vi "read_attributes.vi"(8 "error in (no error)":errorcluster, 11 "CategoricalNB in":refnum<class "CategoricalNB.lvclass">) -> (0 "error out":errorcluster, 2 "attributes":T1, 3 "CategoricalNB out":refnum<class "CategoricalNB.lvclass">)   [LabVIEW 2020, in "CategoricalNB.lvclass"]
uses:
  CategoricalNB.lvclass
  Controls/categorical_nb_attributes.ctl
  CategoricalNB.lvclass/CategoricalNB.ctl
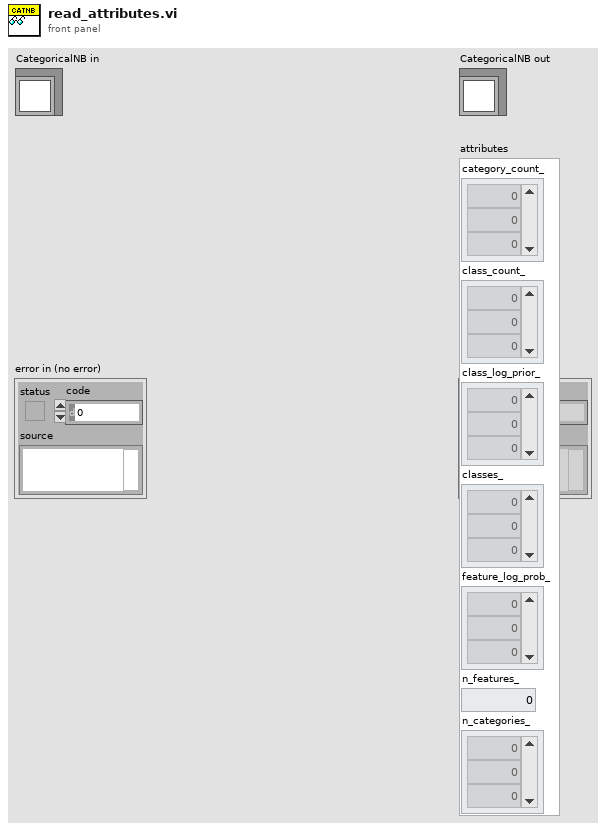
[diagram p1: front panel]
types:
  T1 = typedef "categorical_nb_attributes.ctl" = cluster{"category_count_":dbl[][][], "class_count_":dbl[], "class_log_prior_":dbl[], "classes_":dbl[], "feature_log_prob_":dbl[][][], "n_features_":dbl, "n_categories_":dbl[]}
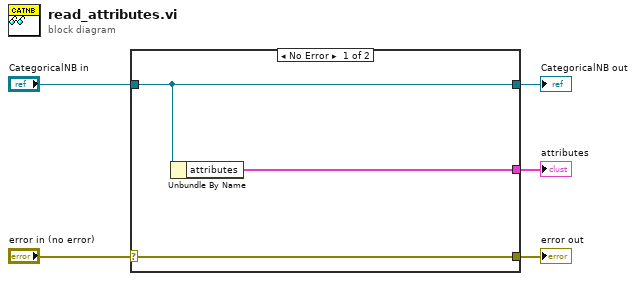
[diagram p0: block diagram]
diagram:
  n1 = case shown="No Error" "error in (no error)" {
    selector: "error in (no error)" -> [w8 w9]
    tunnel: [w8 w9] -> w4
    tunnel: [w7 w10] -> w2
    tunnel: "CategoricalNB in" -> [w7 w10]
    tunnel: [w6 _] -> w1
    frame No Error {
      n2 = Unbundle By Name(w7) -> ("attributes"=w6:T1)
    }
    frame Error {
    }
  }
  "error out" <- w4
  "CategoricalNB out" <- w2
  "attributes" <- w1
